vi "Initialize Attributes Core.vi"(8 "error in (no error)":errorcluster, 10 "Attribute Data":variant, 11 "BNT_DMQmx-MCSV-TC in":refnum<class "BNT_DAQmx-MCSV-RTD.lvclass">) -> (0 "error out":errorcluster, 2 "MandatoryParameters":cluster{"Parameter":string, "found?":bool}[](array[cluster]), 3 "BNT_DMQmx-MCSV-TC out":refnum<class "BNT_DAQmx-MCSV-RTD.lvclass">)   [LabVIEW 2019, in "BNT_DAQmx.lvlib" / "BNT_DAQmx-MCSV-RTD.lvclass"]
doc: "Initialize object attribute.\n\nUnique resources should be allocated elsewhere!"
uses:
  BNT_DAQmx-MCSV-RTD.lvclass
  BNT_DAQmx-MCSV/BNT_DAQmx-MCSV.lvclass
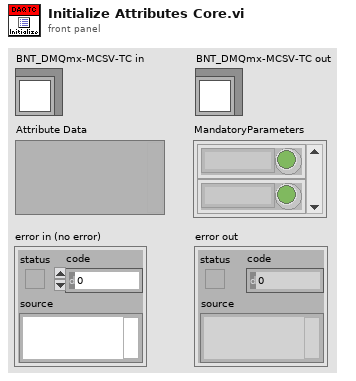
[diagram p1: front panel]
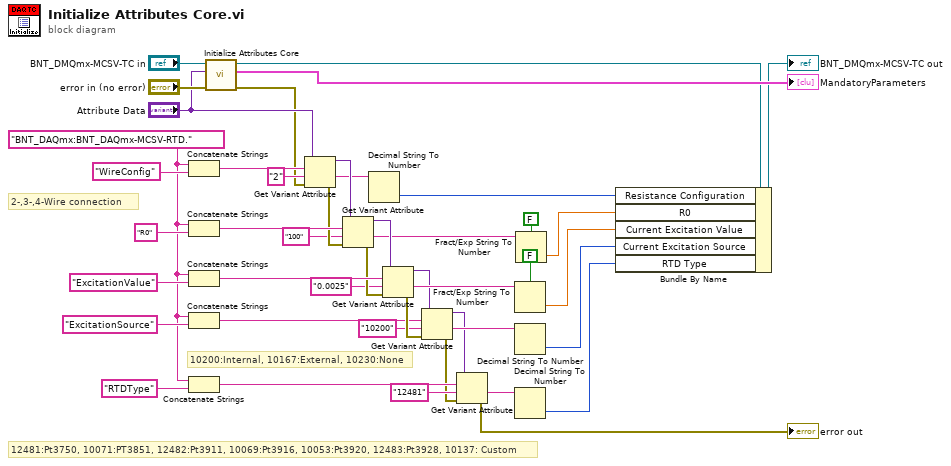
[diagram p0: block diagram]
diagram:
  w6 = "BNT_DAQmx:BNT_DAQmx-MCSV-RTD."
  # "12481:Pt3750, 10071:PT3851, 12482:Pt3911, 10069:Pt3916, 10053:Pt3920, 12483:Pt3928, 10137: Custom"
  # "10200:Internal, 10167:External, 10230:None"
  # "2-,3-,4-Wire connection"
  n1 = Concatenate Strings(w6, "WireConfig" ("string")) -> (w27:string)
  n2 = Concatenate Strings(w6, "R0" ("string")) -> (w38:string)
  n3 = Concatenate Strings(w6, "ExcitationValue" ("string")) -> (w36:string)
  n4 = Concatenate Strings(w6, "ExcitationSource" ("string")) -> (w31:string)
  n5 = Concatenate Strings(w6, "RTDType" ("string")) -> (w8:string)
  n6 = call-parent "Initialize Attributes Core.vi"("error in (no error)"="error in (no error)", "Attribute Data"="Attribute Data", "BNT_DAQmx-MCSV in"="BNT_DMQmx-MCSV-TC in") -> ("error out"=w1:errorcluster, "MandatoryParameters"=→"MandatoryParameters":cluster{"Parameter":string, "found?":bool}[], "BNT_DAQmx-MCSV out"=w23:refnum<class "BNT_DAQmx-MCSV-RTD.lvclass">)  [unwired: 6 in]
  n7 = Get Variant Attribute(Variant="Attribute Data", name=w27, default value (empty Variant)="2", error in=w1) -> (duplicate Variant=w26:variant, value=w21:string, error out=w25:errorcluster)  [unwired: 1 out]
  n8 = Get Variant Attribute(Variant=w26, name=w38, default value (empty Variant)="100", error in=w25) -> (duplicate Variant=w37:variant, value=w12:string, error out=w35:errorcluster)  [unwired: 1 out]
  n9 = Decimal String To Number(string=w21) -> (number=w19:i32)  [unwired: 2 in, 1 out]
  n10 = Get Variant Attribute(Variant=w37, name=w36, default value (empty Variant)="0.0025", error in=w35) -> (duplicate Variant=w32:variant, value=w34:string, error out=w33:errorcluster)  [unwired: 1 out]
  n11 = Get Variant Attribute(Variant=w32, name=w31, default value (empty Variant)="10200", error in=w33) -> (duplicate Variant=w4:variant, value=w30:string, error out=w3:errorcluster)  [unwired: 1 out]
  n12 = Get Variant Attribute(Variant=w4, name=w8, default value (empty Variant)="12481", error in=w3) -> (value=w9:string, error out=→"error out":errorcluster)  [unwired: 2 out]
  n13 = Fract/Exp String To Number(use system decimal point (T)=FALSE, string=w34) -> (number=w17:dbl)  [unwired: 2 in, 1 out]
  n14 = Decimal String To Number(string=w30) -> (number=w15:i32)  [unwired: 2 in, 1 out]
  n15 = Decimal String To Number(string=w9) -> (number=w5:i32)  [unwired: 2 in, 1 out]
  n16 = Fract/Exp String To Number(use system decimal point (T)=FALSE, string=w12) -> (number=w11:dbl)  [unwired: 2 in, 1 out]
  n17 = Bundle By Name(cluster=w23, "Resistance Configuration"=w19, "R0"=w11, "Current Excitation Value"=w17, "Current Excitation Source"=w15, "RTD Type"=w5) -> (→"BNT_DMQmx-MCSV-TC out":refnum<class "BNT_DAQmx-MCSV-RTD.lvclass">)
